vi "Weird Slave.vi"() -> ()   [LabVIEW 2021]
uses:
  API/Slave/Modbus Slave.lvclass
  Transmission Data Unit/ASCII/ASCII Data Unit.lvclass
  Transmission Data Unit/RTU/RTU Data Unit.lvclass
  Network Protocol/Network Slave/TCP/TCP Slave.lvclass
  Data Model/Device Data Model.lvclass
  Transmission Data Unit/IP/IP Data Unit.lvclass
  Data Model/Standard Data Model/Standard Data Model.lvclass
  Transmission Data Unit/Transmission Data Unit.lvclass
  API/Modbus API.lvclass
  Network Protocol/Network Protocol.lvclass
  D:/my_projects/projects/Algorithms/Labview/21/Modbus_v121c/Transmission Data Unit/Transmission Data Unit.lvclass
  D:/my_projects/projects/Algorithms/Labview/21/Modbus_v121c/Transmission Data Unit/IP/IP Data Unit.lvclass
  D:/my_projects/projects/Algorithms/Labview/21/Modbus_v121c/Network Protocol/Network Slave/Network Slave.lvclass
  D:/my_projects/projects/Algorithms/Labview/21/Modbus_v121c/Network Protocol/Network Protocol.lvclass
  D:/my_projects/projects/Algorithms/Labview/21/Modbus_v121c/Network Protocol/Network Slave/TCP/TCP Slave.lvclass
  D:/my_projects/projects/Algorithms/Labview/21/Modbus_v121c/Data Model/Device Data Model.lvclass
  D:/my_projects/projects/Algorithms/Labview/21/Modbus_v121c/Data Model/Standard Data Model/Standard Data Model.lvclass
  D:/my_projects/projects/Algorithms/Labview/21/Modbus_v121c/Transmission Data Unit/Serial Interface/Serial Data Unit.lvclass
  D:/my_projects/projects/Algorithms/Labview/21/Modbus_v121c/Transmission Data Unit/RTU/RTU Data Unit.lvclass
  D:/my_projects/projects/Algorithms/Labview/21/Modbus_v121c/Transmission Data Unit/ASCII/ASCII Data Unit.lvclass
  D:/my_projects/projects/Algorithms/Labview/21/Modbus_v121c/API/Modbus API.lvclass
  D:/my_projects/projects/Algorithms/Labview/21/Modbus_v121c/API/Slave/Modbus Slave.lvclass
  Data Model/Identification Parameters.ctl
  Master Function Definition/Read Device ID code.ctl
panel:
  in  "Port":u16=502
  in  "Serial Type":enum16{"RTU", "ASCII"}(ring)
  in  "Unit ID":u8=1
  in  "HR to write":u16[](array[numeric])=[1, 65535, 40000, 20000]
  in  "Set HR":bool
  in  "Set IR":bool
  in  "IR to write":u16[](array[numeric])=[1, 65535, 40000, 20000]
  in  "IR 6":u16
  in  "Set !":bool
  in  "! status":u8=1
  in  "Set Coils":bool
  in  "Set DI":bool
  in  "DI to write":bool[](array[boolean])=[FALSE, TRUE, FALSE, TRUE]
  in  "coils to write":bool[](array[boolean])=[FALSE, TRUE, FALSE, TRUE]
  in  "set objects":bool
  in  "Objects In":T1[](array[typedef])=[{"Object ID"=0, "Value"="National instruments"}, {"Object ID"=1, "Value"="42"}, {"Object ID"=2, "Value"="1.0.0"}] {"Object ID" format="%x"}
  in  "Coil 6":bool
  out "exception status":u8=1
  out "register values":u16[](array[numeric])=[1, 1, 65535, 40000, 20000, 6]
  out "discrete inputs":bool[](array[boolean])=[FALSE, FALSE, TRUE, FALSE, TRUE, TRUE]
  in  "Read Device ID code":T2
  out "Objects":T1[](array[typedef])=[{"Object ID"=0, "Value"="National instruments"}, {"Object ID"=1, "Value"="42"}, {"Object ID"=2, "Value"="1.0.0"}] {"Object ID" format="%x"}
  in  "Object Id":u8 format="%02x"
  out "holding reg":u16[](array[numeric])=[1, 1, 65535, 40000, 20000, 6]
  out "error out":errorcluster
  in  "stop":bool
  out "Coils":bool[](array[boolean])=[FALSE, FALSE, TRUE, FALSE, TRUE, TRUE] caption="Coils (Master can write coils)"
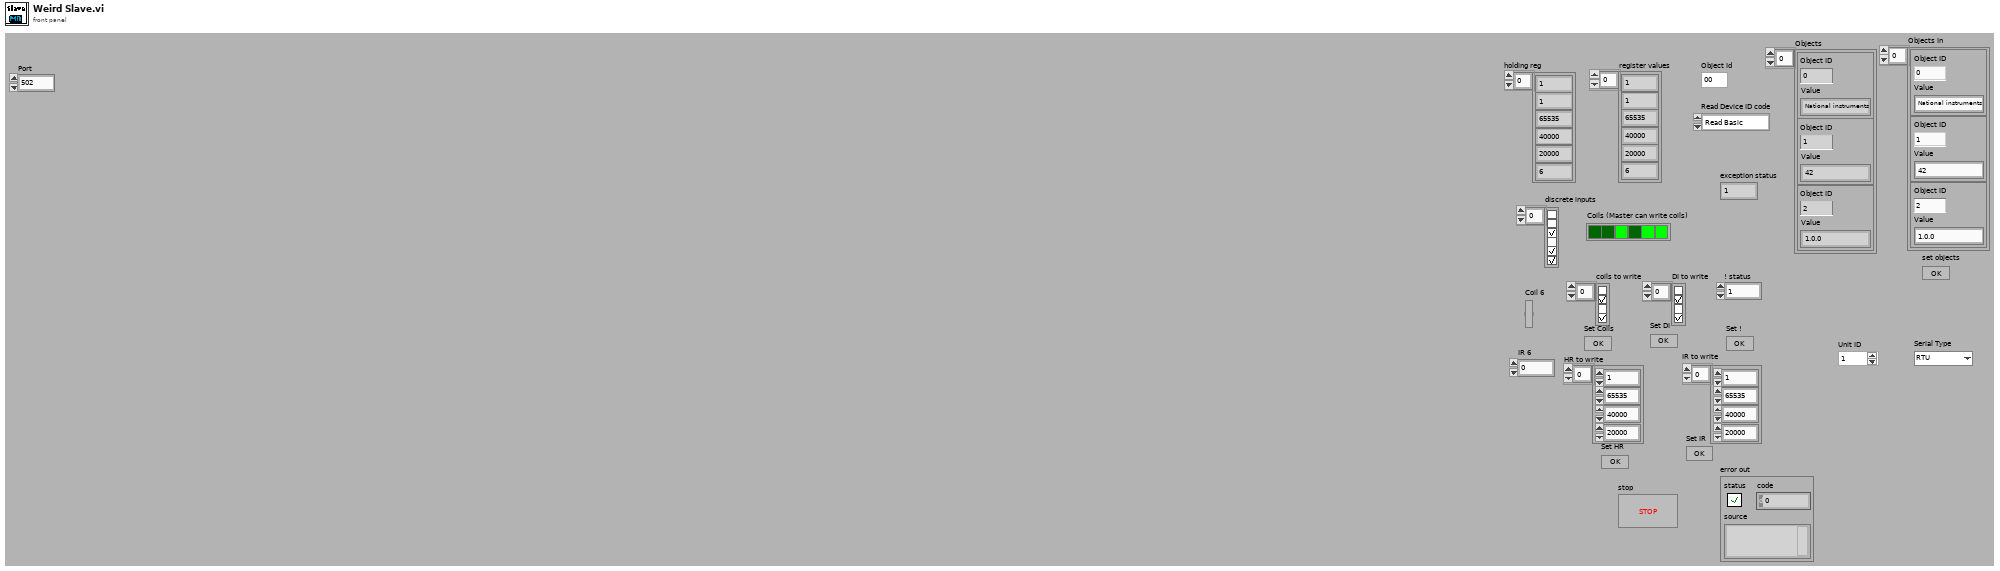
[diagram p1: front panel]
types:
  T1 = typedef "Device Data Model.lvclass/Identification Parameters.ctl" = cluster{"Object ID":u8, "Value":string}
  T2 = typedef "Device Data Model.lvclass/Read Device ID code.ctl" = enum8{"Read Basic", "Read Regular", "Read Extended", "Read Specific"}
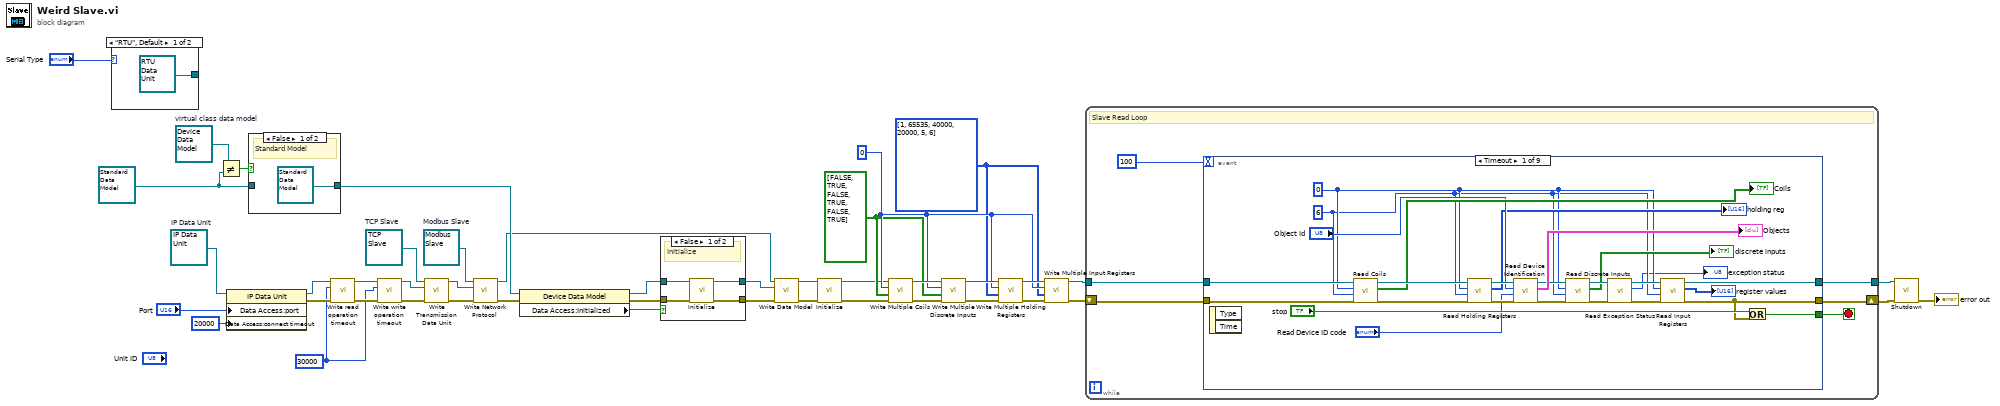
[diagram p0: block diagram]
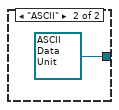
[diagram p4: hidden frame]
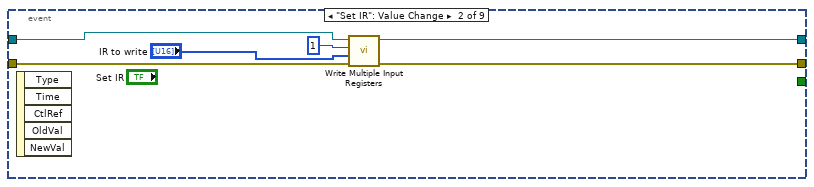
[diagram p5: hidden frame]
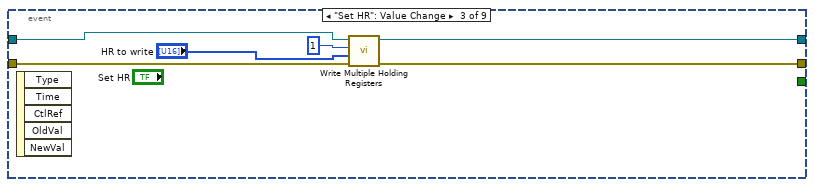
[diagram p6: hidden frame]
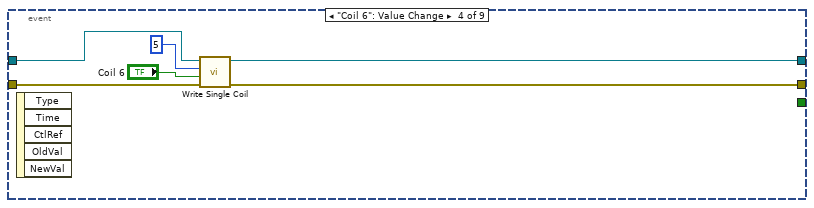
[diagram p7: hidden frame]
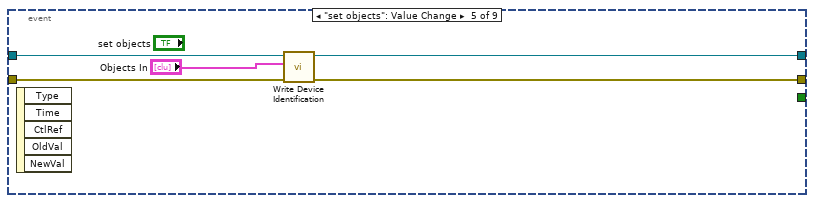
[diagram p8: hidden frame]
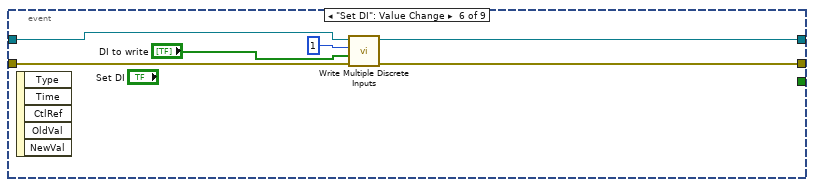
[diagram p9: hidden frame]
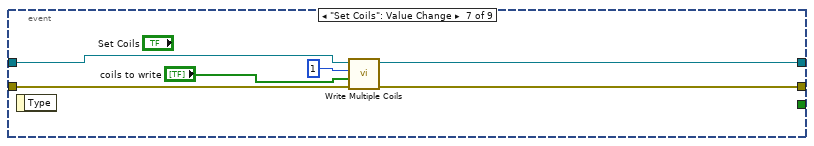
[diagram p10: hidden frame]
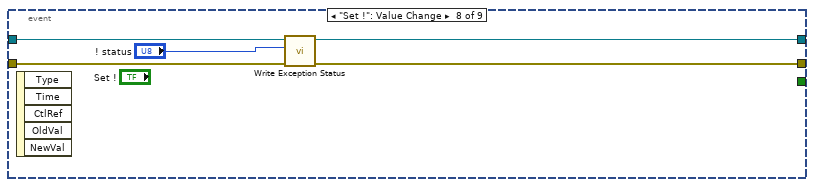
[diagram p11: hidden frame]
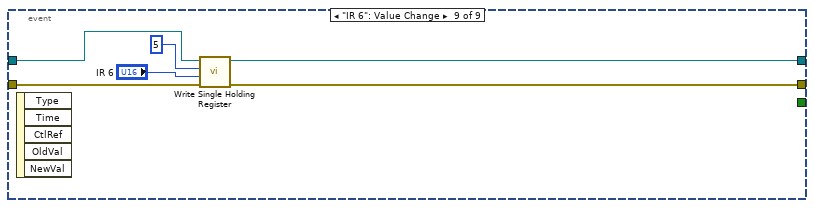
[diagram p12: hidden frame]
diagram:
  w1 = 30000 ("read operation timeout")
  w2 = refnum<class "Standard Data Model.lvclass"> refnum ("Standard Data Model")
  w19 = refnum<class "IP Data Unit.lvclass"> refnum  # IP Data Unit
  w26 = refnum<class "Device Data Model.lvclass"> refnum  # virtual class data model
  w18 = refnum<class "TCP Slave.lvclass"> refnum  # TCP Slave
  w14 = refnum<class "Modbus Slave.lvclass"> refnum  # Modbus Slave
  w31 = bool[] [FALSE, TRUE, FALSE, TRUE, FALSE, TRUE] ("coils to write")
  w32 = u16[] [1, 65535, 40000, 20000, 5, 6] ("registers")
  w33 = u16 0 ("starting address")
  n1 = case shown="\"RTU\", Default" "Serial Type" {
    tunnel: [refnum<class "RTU Data Unit.lvclass"> refnum ("RTU Data Unit") refnum<class "ASCII Data Unit.lvclass"> refnum ("ASCII Data Unit")] -> _
    frame "RTU", Default {
    }
    frame "ASCII" {
    }
  }
  n2 = Not Equal?(x=w26, y=w2) -> (x != y?=w25:bool)
  n3 = property class="IP Data Unit"(reference=w19, "Data Access:port"="Port", "Data Access:connect timeout"=20000 ("connect timeout")) -> (reference out=w7:refnum<class "IP Data Unit.lvclass">, error out=w8:errorcluster)  [unwired: 1 in]
  n4 = case shown="False" w25 {
    tunnel: w2 -> [_ w48]
    tunnel: [refnum<class "Standard Data Model.lvclass"> refnum ("Standard Data Model") w48] -> w24
    frame False {
      # "Standard Model"
    }
    frame True {
    }
  }
  n5 = call "Write read operation timeout.vi"("error in (no error)"=w8, "read operation timeout"=w1, "transmission data unit in"=w7) -> ("error out"=w21:errorcluster, "transmission data unit out"=w20:refnum<class "IP Data Unit.lvclass">)  [unwired: 7 in]
  n6 = call "Write write operation timeout.vi"("error in (no error)"=w21, "write operation timeout"=w1, "transmission data unit in"=w20) -> ("error out"=w10:errorcluster, "transmission data unit out"=w9:refnum<class "IP Data Unit.lvclass">)  [unwired: 7 in]
  n7 = call "Write Transmission Data Unit.vi"("error in (no error)"=w10, "Transmission Data Unit"=w9, "Network Protocol in"=w18) -> ("error out"=w17:errorcluster, "Network Protocol out"=w16:refnum<class "TCP Slave.lvclass">)  [unwired: 7 in]
  n8 = call "Write Network Protocol.vi"("error in (no error)"=w17, "Network Protocol"=w16, "Modbus API in"=w14) -> ("error out"=w15:errorcluster, "Modbus API out"=w13:refnum<class "Modbus Slave.lvclass">)  [unwired: 7 in]
  n9 = property class="Device Data Model"(reference=w24, error in=w15) -> (reference out=w28:refnum<class "Standard Data Model.lvclass">, error out=w29:errorcluster, "Data Access:Initialized"=w27:bool)
  n10 = case shown="False" w27 {
    tunnel: w29 -> [w52 w54]
    tunnel: [w51 w54] -> w22
    tunnel: [w50 w53] -> w23
    tunnel: w28 -> [w49 w53]
    frame False {
      # "Initialize"
      n11 = call-dynamic "Initialize.vi"("error in"=w52, "device data model in"=w49) -> ("error out"=w51:errorcluster, "device data model out"=w50:refnum<class "Standard Data Model.lvclass">)  [unwired: 8 in]
    }
    frame True {
    }
  }
  n12 = call "Write Data Model.vi"("error in (no error)"=w22, "device data model"=w23, "Modbus slave in"=w13) -> ("error out"=w12:errorcluster, "Modbus slave out"=w11:refnum<class "Modbus Slave.lvclass">)  [unwired: 7 in]
  n13 = call-dynamic "Initialize.vi"("error in (no error)"=w12, "Modbus slave in"=w11) -> ("error out"=w4:errorcluster, "Modbus slave out"=w5:refnum<class "Modbus Slave.lvclass">)  [unwired: 8 in]
  n14 = call-dynamic "Write Multiple Coils.vi"("error in (no error)"=w4, "coil values"=w31, "starting address"=w33, "Modbus slave in"=w5) -> ("error out"=w36:errorcluster, "Modbus slave out"=w37:refnum<class "Modbus Slave.lvclass">)  [unwired: 6 in]
  n15 = call-dynamic "Write Multiple Discrete Inputs.vi"("error in (no error)"=w36, "discrete input values"=w31, "starting address"=w33, "Modbus slave in"=w37) -> ("error out"=w39:errorcluster, "Modbus slave out"=w38:refnum<class "Modbus Slave.lvclass">)  [unwired: 6 in]
  n16 = call-dynamic "Write Multiple Holding Registers.vi"("error in (no error)"=w39, "holding register values"=w32, "starting address"=w33, "Modbus slave in"=w38) -> ("error out"=w40:errorcluster, "Modbus slave out"=w41:refnum<class "Modbus Slave.lvclass">)  [unwired: 6 in]
  n17 = call-dynamic "Write Multiple Input Registers.vi"("error in (no error)"=w40, "input register values"=w32, "starting address"=w33, "Modbus slave in"=w41) -> ("error out"=w35:errorcluster, "Modbus slave out"=w34:refnum<class "Modbus Slave.lvclass">)  [unwired: 6 in]
  n18 = while {
    tunnel: [w56] -> w44
    tunnel: w34 -> [w59]
    shift-right: [w57] -> w43
    shift-left: w35 -> [w58]
    stop <- w60 stop-if-true
    # "Slave Read Loop"
    n19 = event shown="[0] Timeout" {
      selector: _ -> [_ _ _ _ _ _ _ _ _]
      dyn-events: _ -> [_ _ _ _ _ _ _ _ _]
      timeout: 100 -> [_ _ _ _ _ _ _ _ _]
      tunnel: [w83 _ _ _ _ _ _ _ _] -> w60
      tunnel: w59 -> [w78 w89 w98 w101 w106 w115 w118 w125 w132]
      tunnel: w58 -> [w77 w90 w95 w102 w107 w114 w119 w126 w131]
      tunnel: [w73 w91 w96 w103 w108 w111 w120 w123 w130] -> w57
      tunnel: [w72 w92 w97 w104 w109 w110 w121 w122 w129] -> w56
      event Timeout {
        w63 = u16 6 ("Number of coils")
        w64 = u16 0 ("Starting Address")
        n20 = event-data() -> ()  [unwired: 1 in, 2 out]
        n21 = call-dynamic "Read Coils.vi"("error in (no error)"=w77, "number of coils"=w63, "starting address"=w64, "Modbus slave in"=w78) -> ("error out"=w82:errorcluster, "coil values"=→"Coils":bool[], "Modbus slave out"=w81:refnum<class "Modbus Slave.lvclass">)  [unwired: 5 in]
        n22 = call-dynamic "Read Holding Registers.vi"("error in (no error)"=w82, "number of holding registers"=w63, "starting address"=w64, "Modbus slave in"=w81) -> ("error out"=w84:errorcluster, "register values"=→"holding reg":u16[], "Modbus slave out"=w85:refnum<class "Modbus Slave.lvclass">)  [unwired: 5 in]
        n23 = call-dynamic "Read Device Identification.vi"("error in (no error)"=w84, "read device ID code"="Read Device ID code", "object ID"="Object Id", "Modbus slave in"=w85) -> ("error out"=w69:errorcluster, "objects"=→"Objects":cluster{"object ID":u8, "value":string}[], "Modbus slave out"=w66:refnum<class "Modbus Slave.lvclass">)  [unwired: 5 in]
        n24 = call-dynamic "Read Discrete Inputs.vi"("error in (no error)"=w69, "number of discrete inputs"=w63, "starting address"=w64, "Modbus slave in"=w66) -> ("error out"=w70:errorcluster, "discrete input values"=→"discrete inputs":bool[], "Modbus slave out"=w68:refnum<class "Modbus Slave.lvclass">)  [unwired: 5 in]
        n25 = call-dynamic "Read Exception Status.vi"("error in (no error)"=w70, "Modbus slave in"=w68) -> ("error out"=w71:errorcluster, "exception status"=→"exception status":u8, "Modbus slave out"=w67:refnum<class "Modbus Slave.lvclass">)  [unwired: 7 in]
        n26 = call-dynamic "Read Input Registers.vi"("error in (no error)"=w71, "number of input registers"=w63, "starting address"=w64, "Modbus slave in"=w67) -> ("error out"=w73:errorcluster, "register values"=→"register values":u16[], "Modbus slave out"=w72:refnum<class "Modbus Slave.lvclass">)  [unwired: 5 in]
        n27 = Or(x="stop", y=w73) -> (x .or. y?=w83:bool)
      }
      event "Set IR": Value Change {
        n28 = event-data() -> ()  [unwired: 1 in, 5 out]
        n29 = call-dynamic "Write Multiple Input Registers.vi"("error in (no error)"=w90, "input register values"="IR to write", "starting address"=u16 1, "Modbus slave in"=w89) -> ("error out"=w91:errorcluster, "Modbus slave out"=w92:refnum<class "Modbus Slave.lvclass">)  [unwired: 6 in]
      }
      event "Set HR": Value Change {
        n30 = event-data() -> ()  [unwired: 1 in, 5 out]
        n31 = call-dynamic "Write Multiple Holding Registers.vi"("error in (no error)"=w95, "holding register values"="HR to write", "starting address"=u16 1, "Modbus slave in"=w98) -> ("error out"=w96:errorcluster, "Modbus slave out"=w97:refnum<class "Modbus Slave.lvclass">)  [unwired: 6 in]
      }
      event "Coil 6": Value Change {
        n32 = event-data() -> ()  [unwired: 1 in, 5 out]
        n33 = call-dynamic "Write Single Coil.vi"("error in (no error)"=w102, "coil value"="Coil 6", "address"=u16 5, "Modbus slave in"=w101) -> ("error out"=w103:errorcluster, "Modbus slave out"=w104:refnum<class "Modbus Slave.lvclass">)  [unwired: 6 in]
      }
      event "set objects": Value Change {
        n34 = event-data() -> ()  [unwired: 1 in, 5 out]
        n35 = call-dynamic "Write Device Identification.vi"("error in (no error)"=w107, "objects"="Objects In", "Modbus slave in"=w106) -> ("error out"=w108:errorcluster, "Modbus slave out"=w109:refnum<class "Modbus Slave.lvclass">)  [unwired: 7 in]
      }
      event "Set DI": Value Change {
        n36 = event-data() -> ()  [unwired: 1 in, 5 out]
        n37 = call-dynamic "Write Multiple Discrete Inputs.vi"("error in (no error)"=w114, "discrete input values"="DI to write", "starting address"=u16 1, "Modbus slave in"=w115) -> ("error out"=w111:errorcluster, "Modbus slave out"=w110:refnum<class "Modbus Slave.lvclass">)  [unwired: 6 in]
      }
      event "Set Coils": Value Change {
        n38 = event-data() -> ()  [unwired: 1 in, 1 out]
        n39 = call-dynamic "Write Multiple Coils.vi"("error in (no error)"=w119, "coil values"="coils to write", "starting address"=u16 1, "Modbus slave in"=w118) -> ("error out"=w120:errorcluster, "Modbus slave out"=w121:refnum<class "Modbus Slave.lvclass">)  [unwired: 6 in]
      }
      event "Set !": Value Change {
        n40 = event-data() -> ()  [unwired: 1 in, 5 out]
        n41 = call "Write Exception Status.vi"("error in (no error)"=w126, "exception status"="! status", "Modbus slave in"=w125) -> ("error out"=w123:errorcluster, "Modbus slave out"=w122:refnum<class "Modbus Slave.lvclass">)  [unwired: 7 in]
      }
      event "IR 6": Value Change {
        n42 = event-data() -> ()  [unwired: 1 in, 5 out]
        n43 = call-dynamic "Write Single Holding Register.vi"("error in (no error)"=w131, "holding register value"="IR 6", "address"=u16 5, "Modbus slave in"=w132) -> ("error out"=w130:errorcluster, "Modbus slave out"=w129:refnum<class "Modbus Slave.lvclass">)  [unwired: 6 in]
      }
    }
  }
  n44 = call-dynamic "Shutdown.vi"("error in (no error)"=w43, "Modbus slave in"=w44) -> ("error out"=→"error out":errorcluster)  [unwired: 9 in]
